vi "Insert Panel To Controller.vi"(0 "Microscope Controller in":refnum<class "Microscope Controller.lvclass">, 5 "Sub Panel":string, 9 "VI Refnum":refnum<vi>, 11 "error in (no error)":errorcluster) -> (4 "Microscope Controller out":refnum<class "Microscope Controller.lvclass">, 15 "error out":errorcluster)   [LabVIEW 2020, in "Microscope.lvlib" / "Microscope Controller.lvlib" / "Microscope Controller.lvclass"]
uses:
  Microscope Controller.lvclass
  Microscope Controller.lvclass/Microscope Controller.ctl
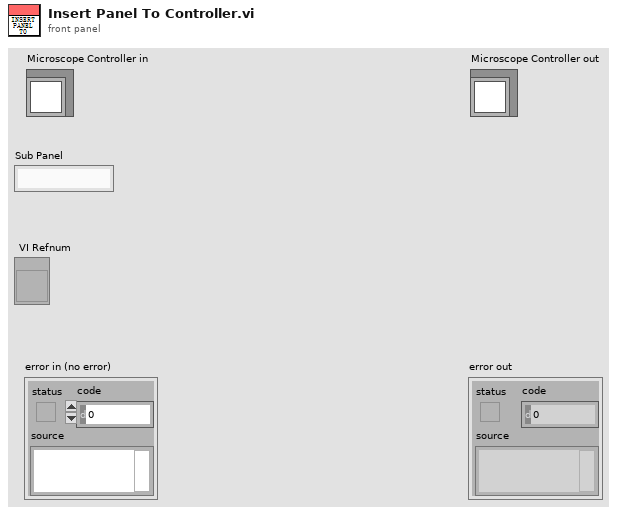
[diagram p1: front panel]
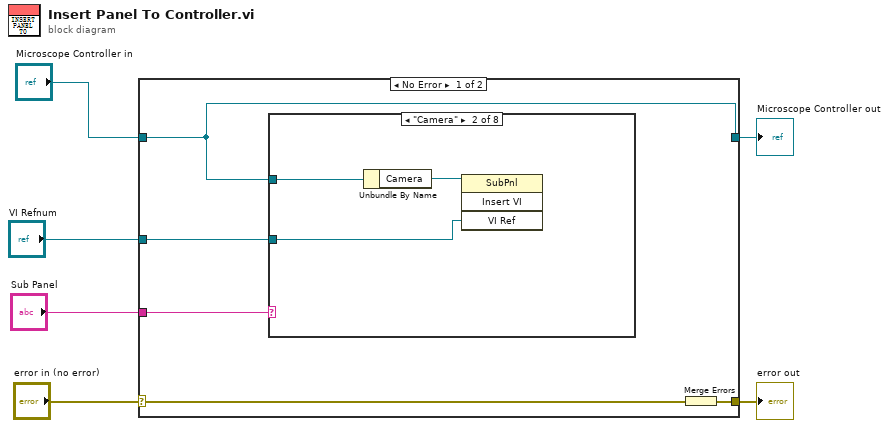
[diagram p0: block diagram]
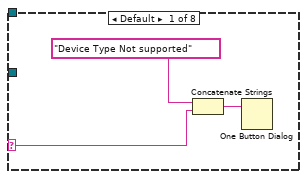
[diagram p2: hidden frame]
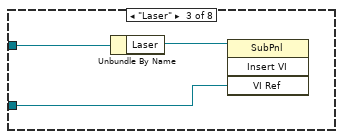
[diagram p3: hidden frame]
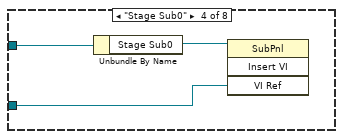
[diagram p4: hidden frame]
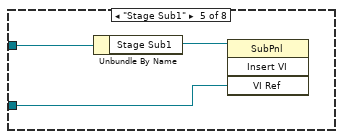
[diagram p5: hidden frame]
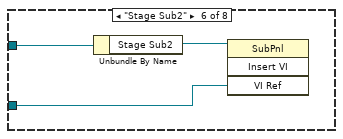
[diagram p6: hidden frame]
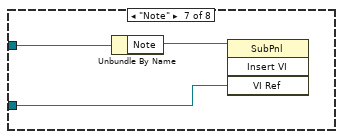
[diagram p7: hidden frame]
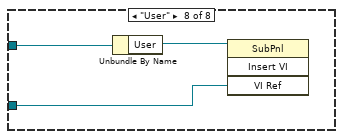
[diagram p8: hidden frame]
diagram:
  n1 = case shown="No Error" "error in (no error)" {
    selector: "error in (no error)" -> [w10 w37]
    tunnel: [w9 w37] -> w5
    tunnel: [w11 w36] -> w3
    tunnel: "Microscope Controller in" -> [w11 w36]
    tunnel: "VI Refnum" -> [w8 _]
    tunnel: "Sub Panel" -> [w7 _]
    frame No Error {
      n2 = case shown="\"Camera\"" w7 {
        selector: w7 -> [w13 _ _ _ _ _ _ _]
        tunnel: w11 -> [_ w17 w20 w23 w26 w29 w32 w35]
        tunnel: w8 -> [_ w15 w18 w21 w24 w27 w30 w33]
        frame Default {
          n3 = Concatenate Strings("Device Type Not supported" ("string"), w13) -> (w14:string)
          n4 = One Button Dialog(message=w14) -> ()  [unwired: 1 in, 1 out]
        }
        frame "Camera" {
          n5 = Unbundle By Name(w17) -> ("Camera"=w16:refnum<vi>)
          n6 = invoke class="SubPnl" method="Insert VI"(reference=w16, "VI Ref"=w15) -> ()  [unwired: 2 in, 4 out]
        }
        frame "Laser" {
          n7 = Unbundle By Name(w20) -> ("Laser"=w19:refnum<vi>)
          n8 = invoke class="SubPnl" method="Insert VI"(reference=w19, "VI Ref"=w18) -> ()  [unwired: 2 in, 4 out]
        }
        frame "Stage Sub0" {
          n9 = Unbundle By Name(w23) -> ("Stage Sub0"=w22:refnum<vi>)
          n10 = invoke class="SubPnl" method="Insert VI"(reference=w22, "VI Ref"=w21) -> ()  [unwired: 2 in, 4 out]
        }
        frame "Stage Sub1" {
          n11 = Unbundle By Name(w26) -> ("Stage Sub1"=w25:refnum<vi>)
          n12 = invoke class="SubPnl" method="Insert VI"(reference=w25, "VI Ref"=w24) -> ()  [unwired: 2 in, 4 out]
        }
        frame "Stage Sub2" {
          n13 = Unbundle By Name(w29) -> ("Stage Sub2"=w28:refnum<vi>)
          n14 = invoke class="SubPnl" method="Insert VI"(reference=w28, "VI Ref"=w27) -> ()  [unwired: 2 in, 4 out]
        }
        frame "Note" {
          n15 = Unbundle By Name(w32) -> ("Note"=w31:refnum<vi>)
          n16 = invoke class="SubPnl" method="Insert VI"(reference=w31, "VI Ref"=w30) -> ()  [unwired: 2 in, 4 out]
        }
        frame "User" {
          n17 = Unbundle By Name(w35) -> ("User"=w34:refnum<vi>)
          n18 = invoke class="SubPnl" method="Insert VI"(reference=w34, "VI Ref"=w33) -> ()  [unwired: 2 in, 4 out]
        }
      }
      n19 = Merge Errors(w10) -> (w9:errorcluster)
    }
    frame Error {
    }
  }
  "error out" <- w5
  "Microscope Controller out" <- w3
